vi "2100_SMU_Meas and Calculate Resitance_Sink Only_No Publish Data.vi"(7 "Current  Level":dbl=-0.01, 8 "error in (no error)":errorcluster, 10 "Pins":string[](array[string]), 11 "Semiconductor Module Context":T1) -> (0 "error Out":errorcluster, 1 "Individial_R_Calc":dbl[](array[numeric]), 2 "R Array":dbl[](array[numeric]), 3 "Semiconductor Module Context Out":T1)   [LabVIEW 2013]
uses:
  <vilib>/NI_TestStand_SemiconductorModule/NI_TestStand_Semiconductor_Module.lvlibp/PinMap/General/SemiconductorModuleContext.ctl
  <vilib>/NI_TestStand_SemiconductorModule/NI_TestStand_Semiconductor_Module.lvlibp/PinMap/DC Power/PinsToNIDCPowerSessions.vi
  <vilib>/NI_TestStand_SemiconductorModule/NI_TestStand_Semiconductor_Module.lvlibp
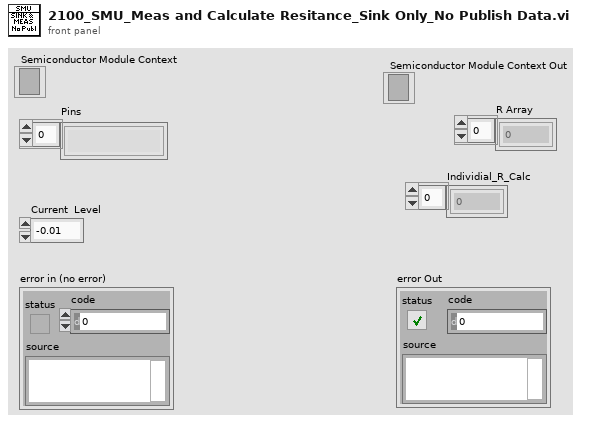
[diagram p1: front panel]
types:
  T1 = typedef "NI_TestStand_Semiconductor_Module.lvlibp/SemiconductorModuleContext.ctl" = refnum<k7>
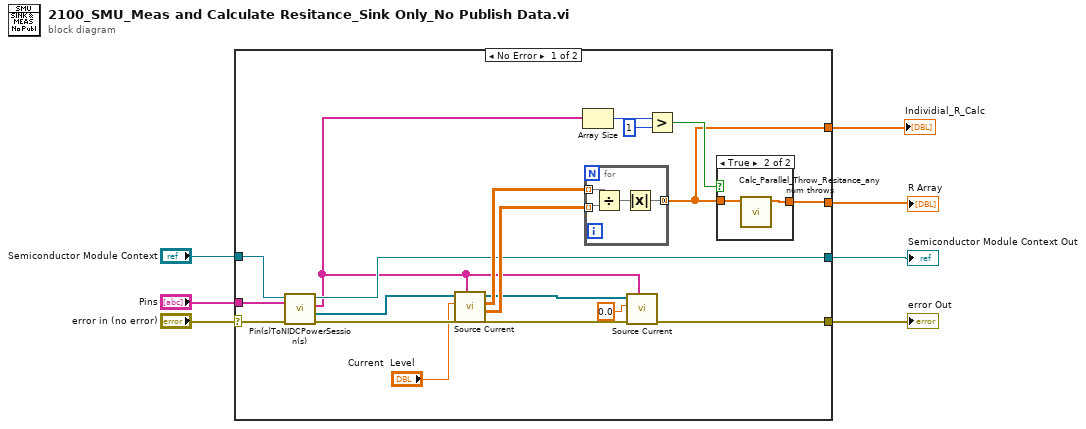
[diagram p0: block diagram]
diagram:
  n1 = case shown="No Error" "error in (no error)" {
    selector: "error in (no error)" -> [w26 w35]
    tunnel: "Semiconductor Module Context" -> [w24 w34]
    tunnel: "Pins" -> [w25 _]
    tunnel: [w15 w35] -> w4
    tunnel: [w14 w34] -> w3
    tunnel: [w13 _] -> w2
    tunnel: [w8 _] -> w1
    frame No Error {
      n2 = call-poly <vilib>:"Pin(s)ToNIDCPowerSession(s).vi"("error in (no error)"=w26, "Pins"=w25, "Semiconductor Module Context"=w24) -> ("error out"=w17:errorcluster, "Instrument Sessions"=w16:refnum<k15>[], "Channel Lists"=w12:string[], "Semiconductor Module Context Out"=w14:T1)  [unwired: 4 in, 1 out]
      n3 = call "Source Current.vi"("Channel Lists"=w12, "error in (no error)"=w17, "current level"="Current  Level", "Instrument Sessions In"=w16) -> ("error out"=w11:errorcluster, "current measurements"=w23:dbl[][], "voltage measurements"=w22:dbl[][], "Instrument Sessions Out"=w10:refnum<k15>[])  [unwired: 4 in]
      n4 = Array Size(array=w12) -> (size(s)=w20:i32)
      n5 = for {
        tunnel: [w32] -> w8 mode=concatenating
        tunnel: w23 -> [w30] mode=indexing
        tunnel: w22 -> [w31] mode=indexing
        n6 = Divide(x=w31, y=w30) -> (x/y=w33:dbl[])
        n7 = Absolute Value(x=w33) -> (abs(x)=w32:dbl[])
      }
      n8 = call "Source Current.vi"("Channel Lists"=w12, "error in (no error)"=w11, "current level"=0.0, "Instrument Sessions In"=w10) -> ("error out"=w15:errorcluster)  [unwired: 4 in, 3 out]
      n9 = Greater?(x=w20, y=1) -> (0:w18:bool)
      n10 = case shown="True" w18 {
        tunnel: w8 -> [w27 w29]
        tunnel: [w27 w28] -> w13
        frame False {
        }
        frame True {
          n11 = call "Calc_Parallel_Throw_Resitance_any num throws.vi"("Resitance_Per Site"=w29) -> ("Parallel_Resitance"=w28:dbl[])  [unwired: 10 in]
        }
      }
    }
    frame Error {
    }
  }
  "error Out" <- w4
  "Semiconductor Module Context Out" <- w3
  "R Array" <- w2
  "Individial_R_Calc" <- w1
